vi "Interpolate 2D.vi"   [LabVIEW 2017, in "NI_Gmath.lvlib"]
doc: "Performs two-dimensional interpolation using a selected interpolation method based on the lookup table defined by <B>X</B>, <B>Y</B>, and <B>Z</B>, where <B>Z</B> is a 2D array. You must manually select the polymorphic instance to use."
uses:
  <vilib>/gmath/NI_Gmath.lvlib
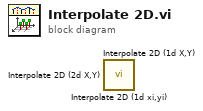
[diagram p0: block diagram]
diagram:
  n1 = call <vilib>:"Interpolate 2D (1d xi,yi).vi"() -> ()  [unwired: 8 in, 4 out]
  n2 = call <vilib>:"Interpolate 2D (1d X,Y).vi"() -> ()  [unwired: 8 in, 4 out]
  n3 = call <vilib>:"Interpolate 2D (2d X,Y).vi"() -> ()  [unwired: 8 in, 4 out]
